vi "many_profiles.vi"() -> ()   [LabVIEW 2013]
panel:
  in  "semester":string(combo)="ws17"
  out "scaling x axis":dbl=0.11695817025440314
  out "max xval":dbl=29.765625 format="%#.1f"
  out "min xval":dbl=-30.0 format="%.1f"
  out "Waveform Graph":dynamicdata(graph)
  in  "common postname":string=".txt"
  in  "common prename":string
  in  "folder":string
  in  "# of files":i32=1
  in  "file names":string[](array[string])=[""]
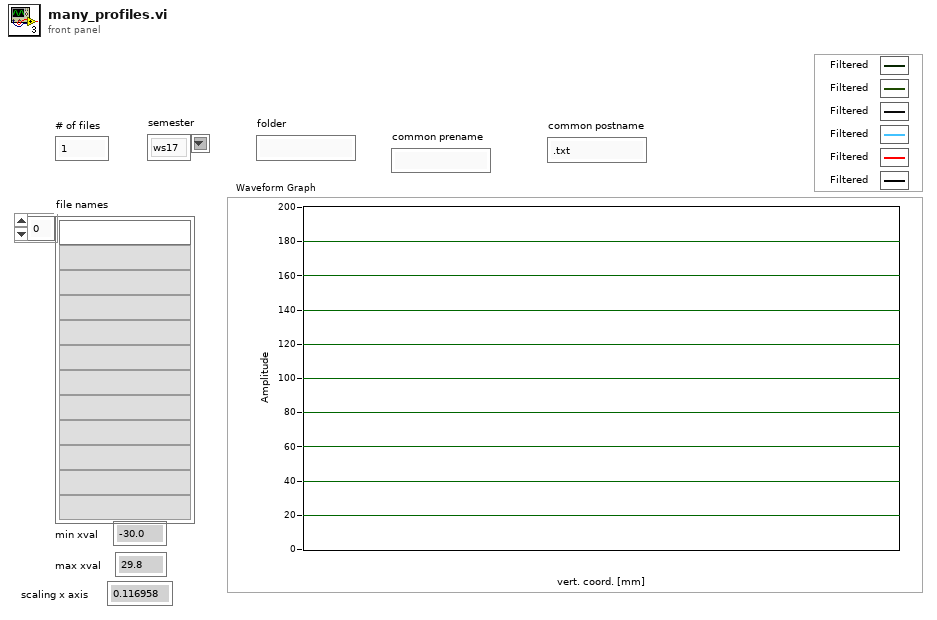
[diagram p1: front panel]
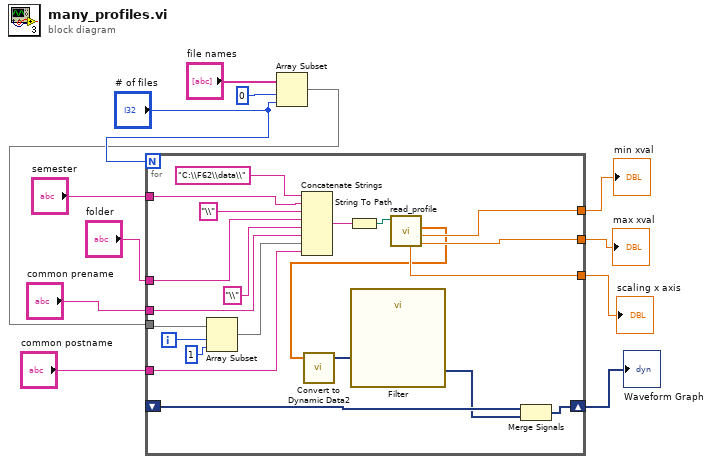
[diagram p0: block diagram]
diagram:
  n1 = Array Subset(array="file names", index=0, length="# of files") -> (w9:string[])
  n2 = for {
    N: "# of files" -> [_]
    tunnel: w9 -> [w33]
    tunnel: "folder" -> [w30]
    tunnel: "common prename" -> [w27]
    tunnel: "common postname" -> [w29]
    shift-right: [w25] -> w5
    shift-left: _ -> [w24]
    tunnel: [w22] -> w4
    tunnel: [w21] -> w3
    tunnel: [w20] -> w2
    tunnel: "semester" -> [w14]
    i -> [w32]
    n3 = Array Subset(array=w33, index=w32, length=1) -> (w28:string[])
    n4 = Concatenate Strings("C:\\F62\\data\\", w14, "\\" ("string"), w30, "\\" ("string"), w27, w28, w29) -> (w13:string)
    n5 = String To Path(string=w13) -> (path=w23:path)
    n6 = call "read_profile.vi"("Path"=w23) -> ("max xval"=w21:dbl, "min xval"=w22:dbl, "yArray"=w19:dbl[], "x/y"=w20:dbl)  [unwired: 6 in, 1 out]
    n7 = call "Convert to Dynamic Data2"("Array"=w19) -> ("Dynamic Data Type"=w18:dynamicdata)  [unwired: 3 in]
    n8 = call "Filter"("Signal"=w18) -> ("Filtered Signal"=w17:dynamicdata)  [unwired: 9 in, 1 out]
    n9 = Merge Signals(w24, w17) -> (w25:dynamicdata)
  }
  "Waveform Graph" <- w5
  "max xval" <- w3
  "min xval" <- w4
  "scaling x axis" <- w2
